vi "Split transient.vi"(5 "Min tw":dbl[unit], 7 "Sampling f":dbl[unit], 8 "Error In":errorcluster, 9 "t in":dbl[](array[numeric]), 10 "Samples in":dbl[](array[numeric])) -> (0 "Error Out":errorcluster, 1 "t out":dbl[](array[numeric]), 2 "Samples out":dbl[](array[numeric]))   [LabVIEW 2019]
doc: "Splits captured data at the capacitance minimum (transient beggining)"
uses:
  <vilib>/Analysis/3filter.llb/Filter Passband Type.ctl
  <vilib>/Analysis/3filter.llb/Butterworth Filter (DBL).vi
  <vilib>/Analysis/NI_AALBase.lvlib
panel:
  out "XY Graph":cluster{"t in":dbl[], "Filtered X":dbl[]}[](graph)
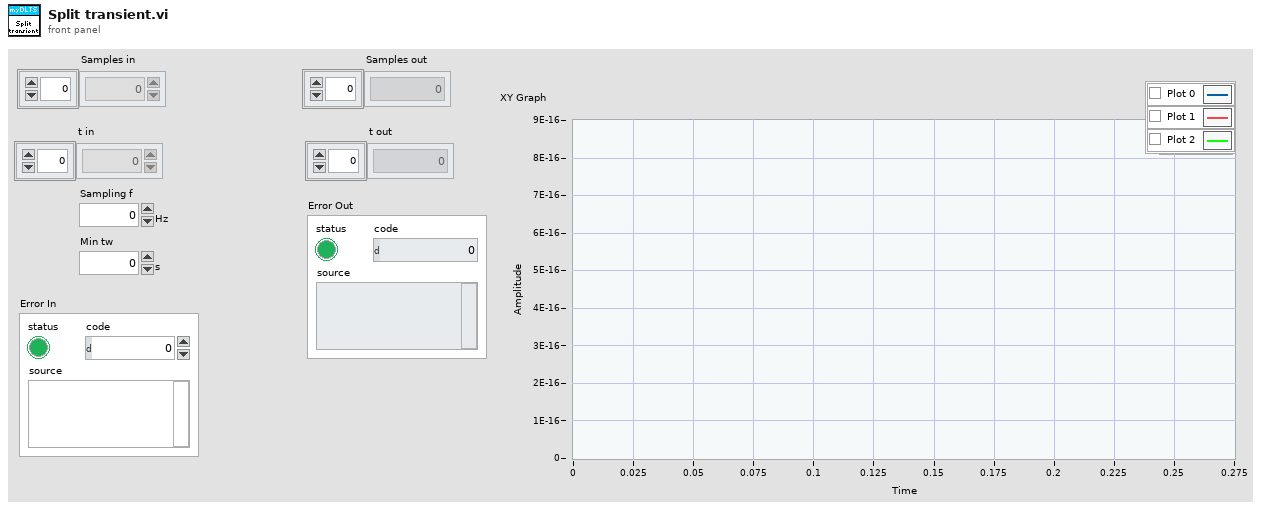
[diagram p1: front panel]
types:
  T1 = typedef "NI_AALBase.lvlib/Filter Passband Type.ctl" = enum32{"Lowpass", "Highpass", "Bandpass", "Bandstop"}
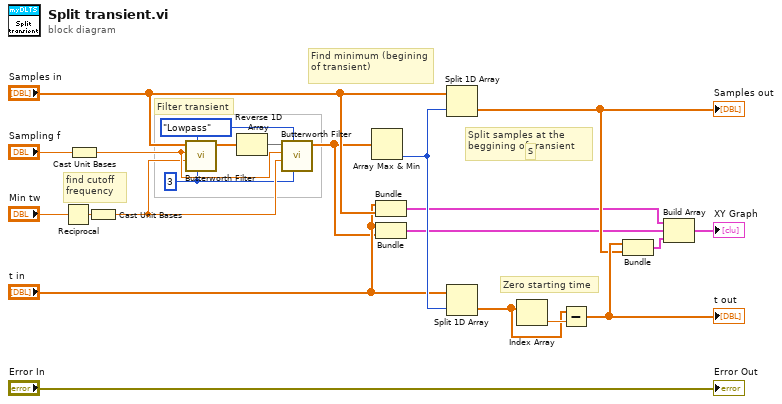
[diagram p0: block diagram]
diagram:
  w1 = 3 ("order")
  w14 = Filter_Passband_Type."Lowpass" ("filter type")
  # "Split samples at the beggining of transient"
  # "Find minimum (begining of transient)"
  # "Filter transient"
  # "find cutoff frequency"
  # "Zero starting time"
  # "S"
  n1 = Reciprocal(x="Min tw") -> (1/x=w11:dbl[unit])
  n2 = Cast Unit Bases(0:"Sampling f") -> (2:w13:dbl)  [unwired: 1 in]
  n3 = Cast Unit Bases(0:w11) -> (2:w12:dbl)  [unwired: 1 in]
  n4 = call-poly <vilib>:"Butterworth Filter.vi"("order"=w1, "filter type"=w14, "high cutoff freq: fh"=w12, "sampling freq: fs"=w13, "X"="Samples in") -> ("Filtered X"=w17:dbl[])  [unwired: 3 in, 1 out]
  n5 = Reverse 1D Array(array=w17) -> (reversed array=w18:dbl[])
  n6 = call-poly <vilib>:"Butterworth Filter.vi"("order"=w1, "filter type"=w14, "high cutoff freq: fh"=w12, "sampling freq: fs"=w13, "X"=w18) -> ("Filtered X"=w8:dbl[])  [unwired: 3 in, 1 out]
  n7 = Array Max & Min(array=w8) -> (min index (indices)=w22:i32)  [unwired: 3 out]
  n8 = Bundle("t in"="t in", "Samples in"="Samples in") -> (w3:cluster{"t in":dbl[], "Samples in":dbl[]})  [unwired: 1 in]
  n9 = Bundle("t in"="t in", "Filtered X"=w8) -> (w4:cluster{"t in":dbl[], "Filtered X":dbl[]})  [unwired: 1 in]
  n10 = Split 1D Array(array="Samples in", index=w22) -> (second subarray=w6:dbl[])  [unwired: 1 out]
  "Samples out" <- w6
  n11 = Split 1D Array(array="t in", index=w22) -> (second subarray=w19:dbl[])  [unwired: 1 out]
  n12 = Index Array(array=w19) -> (element=w20:dbl)  [unwired: 1 in]
  n13 = Subtract(x=w19, y=w20) -> (x-y=w7:dbl[])
  "t out" <- w7
  n14 = Bundle(w7, w6) -> (w5:cluster{dbl[], dbl[]})  [unwired: 1 in]
  n15 = Build Array(w3, w4, w5) -> (→"XY Graph":cluster{"t in":dbl[], "Filtered X":dbl[]}[])
  "Error Out" <- "Error In"
